vi "Test Namer With Shared Approval File Decorating Namer With Folder.vi"(11 "Test Case In":refnum<class "Namer Tests.lvclass">) -> (0 "error out":errorcluster, 3 "Test Case Out":refnum<class "Namer Tests.lvclass">)   [LabVIEW 2020, in "Namer Tests.lvclass"]
uses:
  Namer Tests.lvclass
  C:/Program Files/National Instruments/LabVIEW 2026/vi.lib/Astemes/LUnit/Test Case.lvclass
  Source/Approval Tests/Namer with Folder/Namer with Folder.lvclass
  C:/Users/SAS/Desktop/ApprovalTests.LabVIEW/Source/Approval Tests/Namer/Namer.lvclass
  Source/Approval Tests/Naming Data/Naming Data.lvclass
  Source/Approval Tests/Namer With Shared Approved File/Namer With Shared Approved File.lvclass
  C:/Users/SAS/Desktop/ApprovalTests.LabVIEW/Source/Approval Tests/Namer Decorator/Namer Decorator.lvclass
  Source/Approval Tests/Naming Data/Naming Data.lvclass/Naming Data.ctl
  Source/Approval Tests/Namer With Shared Approved File/Namer With Shared Approved File.lvclass/Namer With Shared Approved File.ctl
  Source/Approval Tests/Namer Decorator/Namer Decorator.lvclass/Namer Decorator.ctl
  <vilib>/Astemes/LUnit/Test Case.lvclass/Test Case.ctl
  4993e8ee-a06a-463a-9684-69129f64d5ce.vi
  52878b9c-9ff9-4b45-a26a-c1090d692375.vi
  Source/Approval Tests/Namer With Shared Approved File/Write Shared Approved File Path.vi
  Source/Approval Tests/Naming Data/Write Test VI Name.vi
  Source/Approval Tests/Naming Data/Write Extension.vi
  Source/Approval Tests/Naming Data/Write Test Label.vi
  Source/Approval Tests/Namer Decorator/Write Decorate.vi
  <vilib>/Astemes/LUnit/Core/LUnit Test Case/Private/Append Pass Result.vi
  <vilib>/Astemes/LUnit/Core/LUnit Test Case/Private/Append Fail Result.vi
  4993e8ee-a06a-463a-9684-69129f64d5ce.vi/9c5d11cd-9439-4240-a1ee-d9baace9c924.vi
  52878b9c-9ff9-4b45-a26a-c1090d692375.vi/9c5d11cd-9439-4240-a1ee-d9baace9c924.vi
  <vilib>/Astemes/LUnit/Core/LUnit Test Case/Private/Run In UI.vi
  <vilib>/Utility/error.llb/Clear Errors.vi
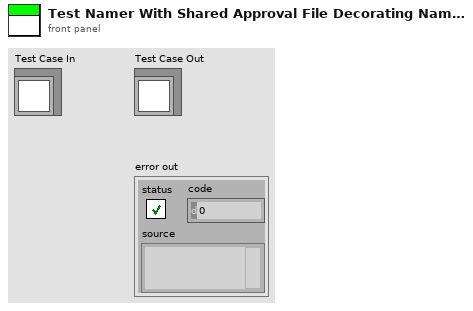
[diagram p1: front panel]
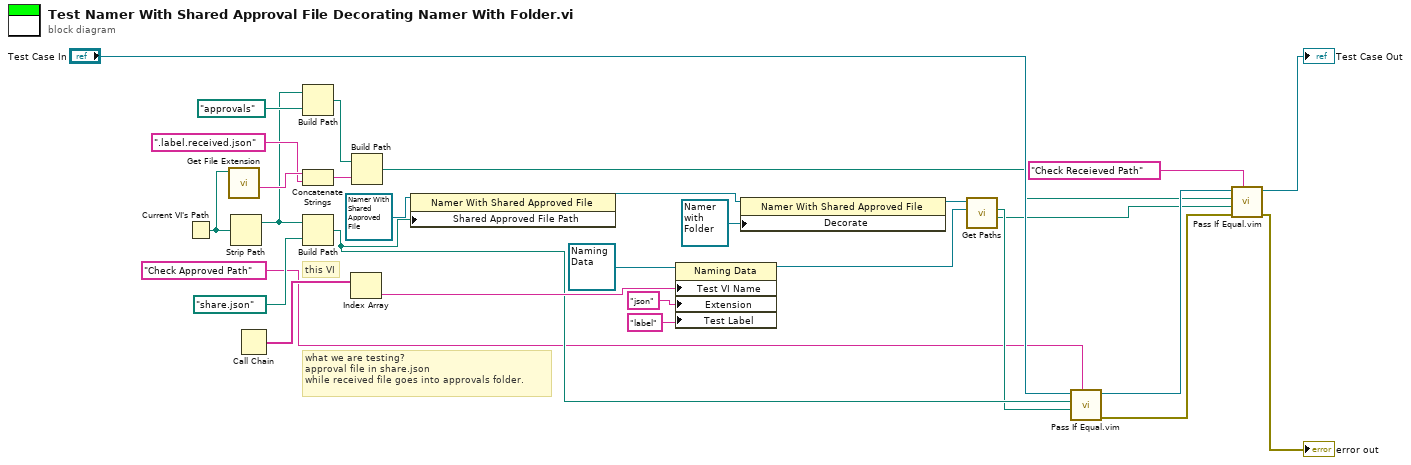
[diagram p0: block diagram]
diagram:
  # "what we are testing?\napproval file in share.json\nwhile received file goes into approvals folder."
  # "this VI"
  n1 = Current VI's Path() -> (path=w22:path)
  n2 = call <vilib>:"Get File Extension.vi"("file"=w22) -> ("filename without extension"=w21:string)  [unwired: 6 in, 4 out]
  n3 = Strip Path(path=w22) -> (stripped path=w10:path)  [unwired: 1 out]
  n4 = Call Chain() -> (call chain=w25:string[])
  n5 = Build Path(base path=w10, name or relative path=path "approvals") -> (appended path=w16:path)
  n6 = Concatenate Strings(w21, ".label.received.json" ("string")) -> (w19:string)
  n7 = Build Path(base path=w10, name or relative path=path "share.json") -> (appended path=w6:path)
  n8 = Index Array(array=w25) -> (element=w24:string)  [unwired: 1 in]
  n9 = Build Path(base path=w16, name or relative path=w19) -> (appended path=w4:path)
  n10 = property on="Property Node" class="Namer With Shared Approved File"(reference=refnum<class "Namer With Shared Approved File.lvclass"> refnum ("Approval Tests:Namer With Shared Approved File.lvclass"), "Shared Approved File Path"=w6) -> (reference out=w11:refnum<class "Namer With Shared Approved File.lvclass">)  [unwired: 1 in, 1 out]
  n11 = property on="Property Node" class="Naming Data"(reference=refnum<class "Naming Data.lvclass"> refnum ("Naming Data"), "Test VI Name"=w24, "Extension"="json", "Test Label"="label") -> (reference out=w23:refnum<class "Naming Data.lvclass">)  [unwired: 1 in, 1 out]
  n12 = property on="Property Node" class="Namer With Shared Approved File"(reference=w11, "Decorate"=refnum<class "Namer with Folder.lvclass"> refnum ("Approval Tests:Namer with SubFolder.lvclass")) -> (reference out=w12:refnum<class "Namer With Shared Approved File.lvclass">)  [unwired: 1 in, 1 out]
  n13 = call-dynamic "Get Paths.vi"("Naming Data"=w23, "Namer With Shared Approved File in"=w12) -> ("Received Path"=w3:path, "Approved Path"=w5:path)  [unwired: 6 in, 2 out]
  n14 = call "Pass If Equal.vim"("Description"="Check Approved Path" ("Label (VI Title)"), "Actual"=w5, "Expected"=w6, "LUnit Test Case In"="Test Case In") -> ("error out"=w28:errorcluster, "LUnit Test Case Out"=w8:refnum<class "Namer Tests.lvclass">)  [unwired: 6 in]
  n15 = call "Pass If Equal.vim"("Description"="Check Receieved Path" ("Label (VI Title)"), "error in (no error)"=w28, "Actual"=w3, "Expected"=w4, "LUnit Test Case In"=w8) -> ("error out"=→"error out":errorcluster, "LUnit Test Case Out"=→"Test Case Out":refnum<class "Namer Tests.lvclass">)  [unwired: 5 in]
